vi "Invert Relay.vi"(4 "Simulate":bool, 6 "timeout":dbl=10.0 format="%0.2f", 8 "error in":errorcluster, 11 "DO-Line Ref":refnum<k21>) -> (0 "error out":errorcluster, 3 "DO-Line Ref out":refnum<k21>)   [LabVIEW 2022 SP3, in "DAQ.lvclass"]
doc: "Developed by Kevin Thompson\nkevin@thompsonengineering.net\n\nCopyright 2018-2020\nThompson Engineering, LLC"
uses:
  DAQ.lvclass
  DAQ.lvclass/DAQ.ctl
  <vilib>/DAQmx/read.llb/DAQmx Read (Digital Bool 1Line 1Point).vi
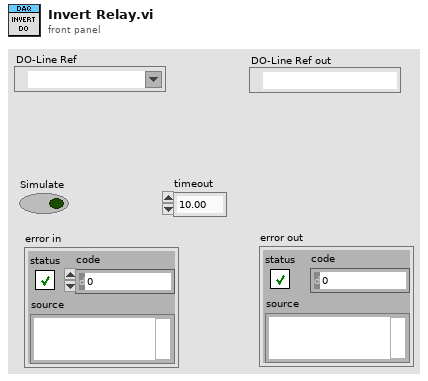
[diagram p1: front panel]
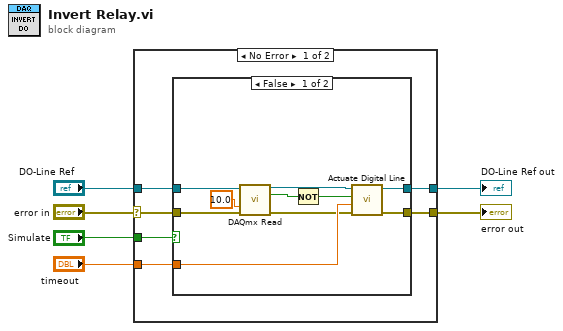
[diagram p0: block diagram]
diagram:
  n1 = case shown="No Error" "error in" {
    selector: "error in" -> [w10 w26]
    tunnel: "DO-Line Ref" -> [w12 w25]
    tunnel: [w11 w26] -> w5
    tunnel: [w9 w25] -> w3
    tunnel: "timeout" -> [w8 _]
    tunnel: "Simulate" -> [w7 _]
    frame No Error {
      n2 = case shown="False" w7 {
        tunnel: w12 -> [w18 w24]
        tunnel: [w22 w23] -> w11
        tunnel: w10 -> [w13 w23]
        tunnel: [w21 w24] -> w9
        tunnel: w8 -> [w20 _]
        frame False {
          n3 = call-poly <vilib>:"DAQmx Read.vi"("task/channels in"=w18, "timeout"=10.0, "error in"=w13) -> ("task out"=w17:refnum<k21>, "data"=w16:bool, "error out"=w14:errorcluster)  [unwired: 10 in]
          n4 = Not(x=w16) -> (.not. x?=w15:bool)
          n5 = call "Actuate Digital Line.vi"("error in"=w14, "timeout"=w20, "state"=w15, "DO-Line Ref"=w17) -> ("error out"=w22:errorcluster, "DO-Line Ref out"=w21:refnum<k21>)  [unwired: 6 in]
        }
        frame True {
        }
      }
    }
    frame Error {
    }
  }
  "error out" <- w5
  "DO-Line Ref out" <- w3
